vi "Actor Core.vi"(8 "error in":errorcluster, 11 "HIJ Vision Launcher in":refnum<class "HIJ Vision Launcher.lvclass">) -> (0 "error out":errorcluster, 3 "Actor out":refnum<class "Actor.lvclass">)   [LabVIEW 2020, in "HIJ Vision Launcher.lvlib" / "HIJ Vision Launcher.lvclass"]
doc: "(<B>Filename</B>: Actor Framework.lvlib:Actor.lvclass:Actor Core.vi)\n\nReceives messages to the actor, reacts to them, and initiates any error handling that may shut the actor down.\n\nDescendant classes may override this VI to append parallel tasks for the actor to complete while it handles messages. Overrides use the Call Parent Method node."
uses:
  HIJ Vision Launcher.lvclass
  C:/POLARIS Programme/POLARIS-AS-3-Cams/Submodules/Viewable Actor/ViewableActorEncaps/ViewableActorEncaps.lvclass
  C:/POLARIS Programme/POLARIS-AS-3-Cams/Submodules/Viewable Actor/ViewableActor/ViewableActor.lvclass
  C:/Program Files (x86)/National Instruments/LabVIEW 2020/vi.lib/ActorFramework/Actor/Actor.lvclass
  <vilib>/ActorFramework/Actor/Actor.lvclass
  <vilib>/userdefined/High Color/IMAQdx.ctl
  HIJ Vision Launcher.lvclass/HIJ Vision Launcher.ctl
  Viewable Actor/ViewableActor/ViewableActor.lvclass/ViewableActor.ctl
  <vilib>/ActorFramework/Actor/Actor.lvclass/Actor.ctl
  <vilib>/ActorFramework/Message Enqueuer/Message Enqueuer.lvclass/Message Enqueuer.ctl
  Start Parameter.ctl
  HIJ Vision Launcher Messages/Set Start Parameter Msg/Set Start Parameter Msg.lvclass/Set Start Parameter Msg.ctl
  <vilib>/ActorFramework/Report Error Msg/Report Error Msg.lvclass/Report Error Msg.ctl
  Read Cmd Parameters.vi
  Viewable Actor/ViewableActor/Read Config URL.vi
  <vilib>/ActorFramework/Message Enqueuer/Init from Existing Queue.vi
  <vilib>/ActorFramework/Message Enqueuer/Enqueue.vi
  HIJ Vision Launcher Messages/Set Start Parameter Msg/Set Start Parameter Msg.lvclass
  C:/Program Files (x86)/National Instruments/LabVIEW 2020/vi.lib/ActorFramework/Message/Message.lvclass
  HIJ Vision Launcher Messages/Launch Application Msg/Launch Application Msg.lvclass
  <vilib>/ActorFramework/Stop Msg/Stop Msg.lvclass
  <vilib>/ActorFramework/Report Error Msg/Report Error Msg.lvclass
  <vilib>/Utility/config.llb/Read Key (Path).vi
  <vilib>/Utility/config.llb/Read Key (String).vi
  <vilib>/ActorFramework/Message Priority Queue/Priority Enqueue.vi
  <vilib>/Utility/config.llb/Write Key (Path).vi
  <vilib>/Utility/config.llb/Write Key (String).vi
  <vilib>/ActorFramework/Message Enqueuer/Message Enqueuer.lvclass
  Viewable Actor/ViewableActorEncaps/ViewableActorEncaps.lvclass
  <vilib>/Utility/config.llb/NI_LVConfig.lvlib
panel:
  in  "Camera":T1="TestCam"
  in  "Windows Titel":string
  in  "Camera ConfigDir":path=path "C:/Users/user/Desktop/test/ConfigDir"
  in  "Start WorkDir":path=path "C:/Users/user/Desktop/test/WorkDir"
  in  "Stop Signal":bool
  in  "RUN_STOP":bool
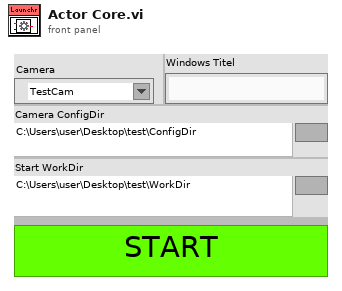
[diagram p1: front panel]
types:
  T1 = typedef "IMAQdx.ctl" = refnum<k21>
  T2 = typedef "HIJ Vision Launcher.lvlib/HIJ Vision Launcher.lvclass/Start Parameter.ctl" = cluster{"Windows Titel":string, "Start WorkDir":path, "Camera ConfigDir":path, "Camera":T1}
  T3 = typedef "NI_LVConfig.lvlib/Config Data RefNum.ctl" = refnum<k1>
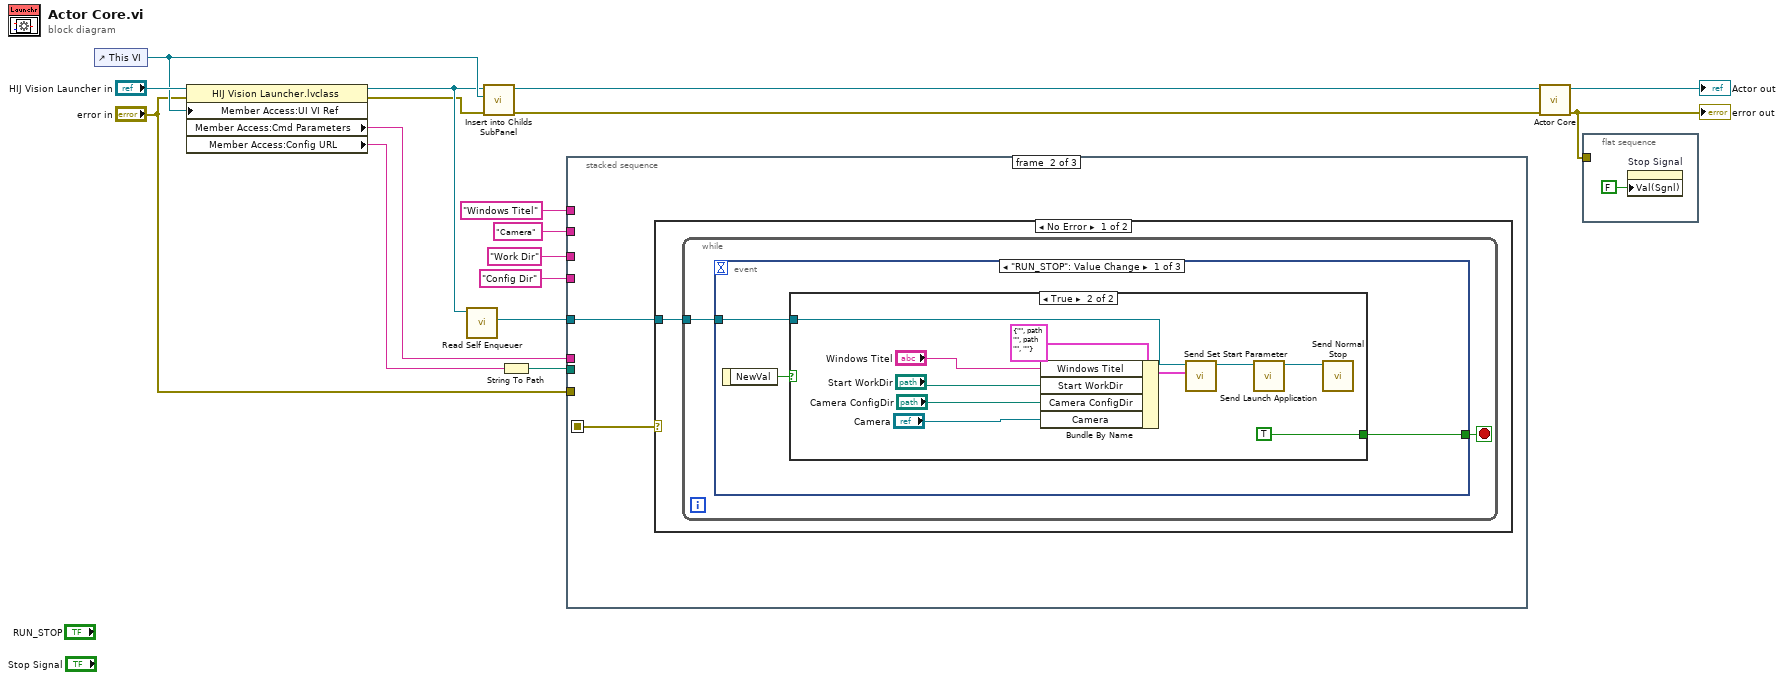
[diagram p0: block diagram]
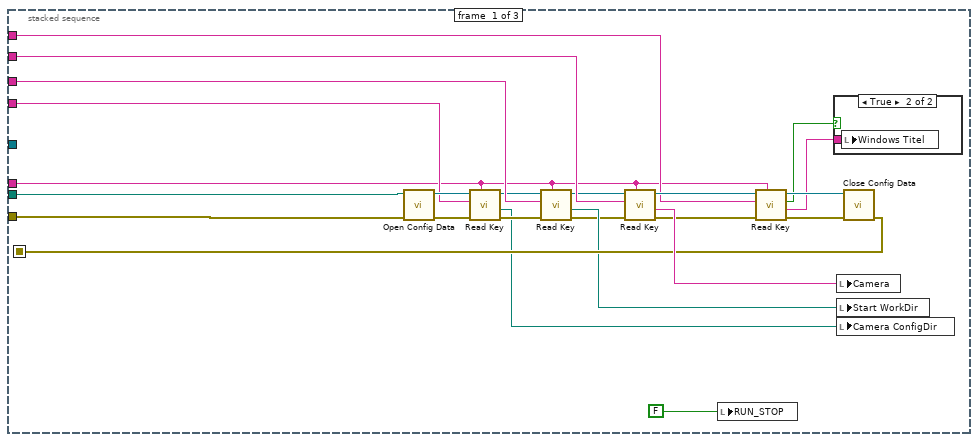
[diagram p2: hidden frame]
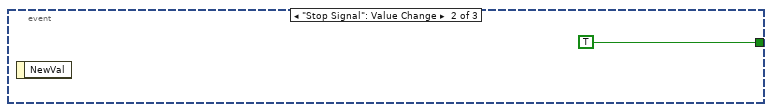
[diagram p5: hidden frame]
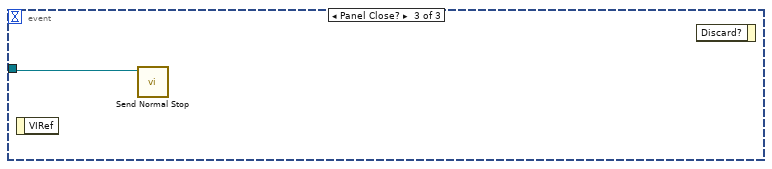
[diagram p6: hidden frame]
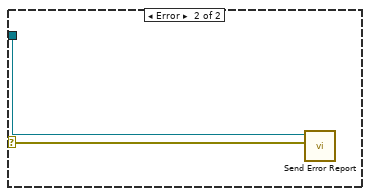
[diagram p7: hidden frame]
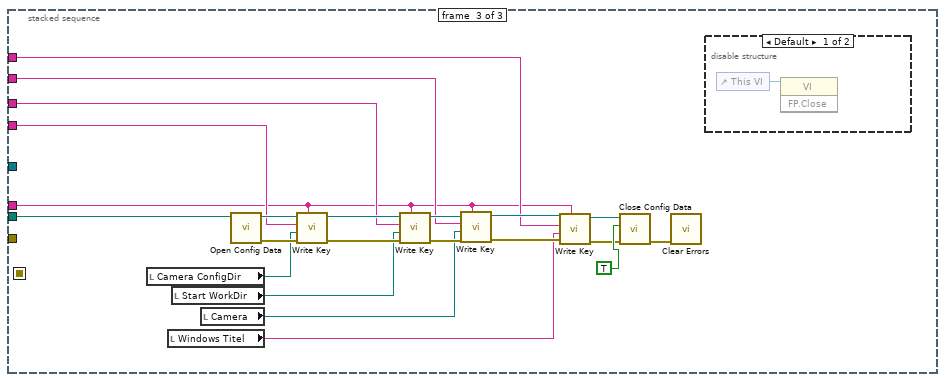
[diagram p8: hidden frame]
diagram:
  n1 = control-ref of="This VI"() -> (w14:refnum<vi>)
  n2 = property class="HIJ Vision Launcher.lvclass"(reference="HIJ Vision Launcher in", error in="error in", "Member Access:UI VI Ref"=w14) -> (reference out=w8:refnum<class "HIJ Vision Launcher.lvclass">, error out=w5:errorcluster, "Member Access:Cmd Parameters"=w1:string, "Member Access:Config URL"=w2:string)
  n3 = call <vilib>:"Read Self Enqueuer.vi"("Actor"=w8) -> ("Self Enqueuer"=w7:refnum<class "Message Enqueuer.lvclass">)  [unwired: 10 in]
  n4 = call-dynamic "Insert into Childs SubPanel.vi"("error in (no error)"=w5, "UI VI Ref"=w14, "ViewableActorEncaps in"=w8) -> ("error out"=w4:errorcluster, "ViewableActorEncaps out"=w15:refnum<class "HIJ Vision Launcher.lvclass">)  [unwired: 7 in]
  n5 = String To Path(string=w2) -> (path=w3:path)
  n6 = stacked-sequence {
    seq-local: [w37 _ _] -> [_ w44 _]
    tunnel: "Config Dir" ("key") -> [w38 _ w84]
    tunnel: "Work Dir" ("key") -> [w36 _ w75]
    tunnel: "Camera" ("key") -> [w35 _ w74]
    tunnel: "Windows Titel" ("key") -> [w25 _ w67]
    tunnel: "error in" -> [w21 _ _]
    tunnel: w7 -> [_ w43 _]
    tunnel: w3 -> [w19 _ w65]
    tunnel: w1 -> [w18 _ w66]
    frame #0 {
      n7 = call <vilib>:"Open Config Data.vi"("error in (no error)"=w21, "configuration file path"=w19) -> ("error out"=w40:errorcluster, "refnum"=w39:T3)  [unwired: 7 in, 1 out]
      n8 = call-poly <vilib>:"Read Key.vi"("section"=w18, "error in (no error)"=w40, "key"=w38, "refnum"=w39) -> ("error out"=w33:errorcluster, "value"=w30:path, "refnum out"=w34:T3)  [unwired: 4 in, 1 out]
      n9 = call-poly <vilib>:"Read Key.vi"("section"=w18, "error in (no error)"=w33, "key"=w36, "refnum"=w34) -> ("error out"=w27:errorcluster, "value"=w29:path, "refnum out"=w28:T3)  [unwired: 4 in, 1 out]
      n10 = call-poly <vilib>:"Read Key.vi"("section"=w18, "error in (no error)"=w27, "key"=w35, "refnum"=w28) -> ("error out"=w24:errorcluster, "value"=w41:string, "refnum out"=w32:T3)  [unwired: 4 in, 1 out]
      n11 = local write "RUN_STOP"(FALSE ("RUN_STOP")) -> ()
      n12 = call-poly <vilib>:"Read Key.vi"("section"=w18, "error in (no error)"=w24, "key"=w25, "refnum"=w32) -> ("error out"=w23:errorcluster, "value"=w22:string, "found?"=w20:bool, "refnum out"=w26:T3)  [unwired: 4 in]
      n13 = case shown="True" w20 {
        tunnel: w22 -> [_ w42]
        frame False {
        }
        frame True {
          n14 = local write "Windows Titel"(w42) -> ()
        }
      }
      n15 = local write "Camera"(w41) -> ()
      n16 = local write "Start WorkDir"(w29) -> ()
      n17 = local write "Camera ConfigDir"(w30) -> ()
      n18 = call <vilib>:"Close Config Data.vi"("error in (no error)"=w23, "refnum"=w26) -> ("error out"=w37:errorcluster)  [unwired: 8 in, 1 out]
    }
    frame #1 {
      n19 = case shown="No Error" w44 {
        selector: w44 -> [_ w63]
        tunnel: w43 -> [w45 w64]
        frame No Error {
          n20 = while {
            tunnel: w45 -> [w46]
            stop <- w47 stop-if-true
            n21 = event shown="[0] \"RUN_STOP\": Value Change" {
              selector: _ -> [_ _ _]
              dyn-events: _ -> [_ _ _]
              timeout: _ -> [_ _ _]
              tunnel: [w50 TRUE _] -> w47
              tunnel: w46 -> [w48 _ w62]
              event "RUN_STOP": Value Change {
                n22 = event-data() -> ("NewVal"=w49:bool)  [unwired: 1 in]
                n23 = case shown="True" w49 {
                  tunnel: [_ TRUE] -> w50
                  tunnel: w48 -> [_ w59]
                  frame False {
                  }
                  frame True {
                    n24 = Bundle By Name(cluster=T2 {"Windows Titel"="", "Start WorkDir"=path "", "Camera ConfigDir"=path "", "Camera"=""} ("Start Parameter"), "Windows Titel"="Windows Titel", "Start WorkDir"="Start WorkDir", "Camera ConfigDir"="Camera ConfigDir", "Camera"="Camera") -> (w56:T2)
                    n25 = call "Send Set Start Parameter.vi"("Start Parameter"=w56, "Message Enqueuer"=w59) -> ("Message Enqueuer out"=w58:refnum<class "Message Enqueuer.lvclass">)  [unwired: 8 in, 1 out]
                    n26 = call "Send Launch Application.vi"("Message Enqueuer"=w58) -> ("Message Enqueuer out"=w51:refnum<class "Message Enqueuer.lvclass">)  [unwired: 9 in, 1 out]
                    n27 = call <vilib>:"Send Normal Stop.vi"("Message Enqueuer"=w51) -> ()  [unwired: 10 in, 1 out]
                  }
                }
              }
              event "Stop Signal": Value Change {
                n28 = event-data() -> ()  [unwired: 1 in, 1 out]
              }
              event Panel Close? {
                n29 = event-data() -> ()  [unwired: 1 in, 1 out]
                n30 = call <vilib>:"Send Normal Stop.vi"("Message Enqueuer"=w62) -> ()  [unwired: 10 in, 1 out]
                n31 = event-data() -> ()  [unwired: 2 in, 1 out]
              }
            }
          }
        }
        frame Error {
          n32 = call <vilib>:"Send Error Report.vi"("Error From Sender"=w63, "Message Enqueuer"=w64) -> ()  [unwired: 9 in, 1 out]
        }
      }
    }
    frame #2 {
      n33 = local read "Camera ConfigDir"() -> (w77:path)
      n34 = local read "Windows Titel"() -> (w68:string)
      n35 = local read "Start WorkDir"() -> (w76:path)
      n36 = local read "Camera"() -> (w73:T1)
      n37 = call <vilib>:"Open Config Data.vi"("configuration file path"=w65) -> ("error out"=w83:errorcluster, "refnum"=w85:T3)  [unwired: 8 in, 1 out]
      n38 = call-poly <vilib>:"Write Key.vi"("section"=w66, "error in (no error)"=w83, "value"=w77, "key"=w84, "refnum"=w85) -> ("error out"=w82:errorcluster, "refnum out"=w86:T3)  [unwired: 4 in, 1 out]
      n39 = call-poly <vilib>:"Write Key.vi"("section"=w66, "error in (no error)"=w82, "value"=w76, "key"=w75, "refnum"=w86) -> ("error out"=w78:errorcluster, "refnum out"=w79:T3)  [unwired: 4 in, 1 out]
      n40 = call-poly <vilib>:"Write Key.vi"("section"=w66, "error in (no error)"=w78, "value"=w73, "key"=w74, "refnum"=w79) -> ("error out"=w70:errorcluster, "refnum out"=w72:T3)  [unwired: 4 in, 1 out]
      n41 = call-poly <vilib>:"Write Key.vi"("section"=w66, "error in (no error)"=w70, "value"=w68, "key"=w67, "refnum"=w72) -> ("error out"=w69:errorcluster, "refnum out"=w71:T3)  [unwired: 4 in, 1 out]
      n42 = call <vilib>:"Close Config Data.vi"("error in (no error)"=w69, "write file if changed (T)"=TRUE, "refnum"=w71) -> ("error out"=w81:errorcluster)  [unwired: 7 in, 1 out]
      n43 = call <vilib>:"Clear Errors.vi"("error in (no error)"=w81) -> ()  [unwired: 5 in, 2 out]
      n44 = disable-structure shown="Default" {
        frame condition #0 {
          n45 = control-ref of="This VI"() -> (w87:refnum<vi>)
          n46 = invoke class="VI" method="FP.Close"(reference=w87) -> ()  [unwired: 2 in, 3 out]
        }
        frame condition #1 (active) {
        }
      }
    }
  }
  n47 = call-parent "Actor Core.vi"("error in"=w4, "Actor in"=w15) -> ("error out"=w6:errorcluster, "Actor out"=→"Actor out":refnum<class "Actor.lvclass">)  [unwired: 8 in]
  "error out" <- w6
  n48 = flat-sequence {
    tunnel: w6 -> [_]
    frame #0 {
      n49 = property on="Stop Signal" class="Bool (strict)"("Val(Sgnl)"=FALSE ("Value (Signaling)")) -> ()  [unwired: 2 in, 2 out]
    }
  }
